vi "Timeout Topics (Global).vi"() -> ()   [LabVIEW 2018]
panel:
  in  "Timeout Gen":bool
  in  "Timeout ES2":bool
  in  "Timeout ES1":bool
  in  "Timeout PV":bool
  in  "Timeout PCC":bool
  in  "Timeout Load":bool
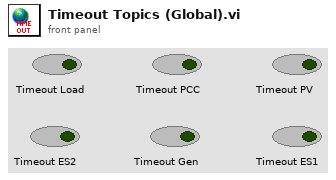
[diagram p1: front panel]
diagram:
